vi "ENA_Recall Inst Setup.vi"(0 "Semiconductor Module Context":T1, 5 "Pins":string[](array[string])=["RF1", "RF2"], 11 "error in (no error)":errorcluster) -> (6 "Semiconductor Module Context Out":T1, 15 "error out":errorcluster)   [LabVIEW 2013]
uses:
  <vilib>/NI_TestStand_SemiconductorModule/NI_TestStand_Semiconductor_Module.lvlibp/PinMap/General/SemiconductorModuleContext.ctl
  Pin Map API/ENA Custom Instrument.lvlib
  <vilib>/NI_TestStand_SemiconductorModule/NI_TestStand_Semiconductor_Module.lvlibp
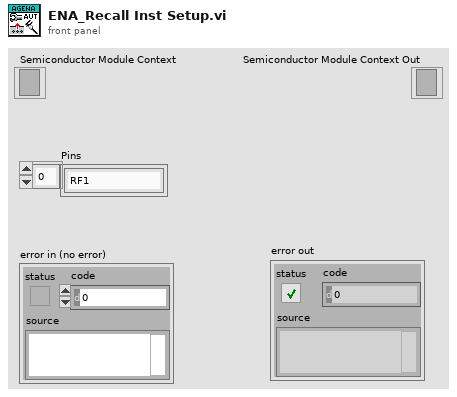
[diagram p1: front panel]
types:
  T1 = typedef "NI_TestStand_Semiconductor_Module.lvlibp/SemiconductorModuleContext.ctl" = refnum<k7>
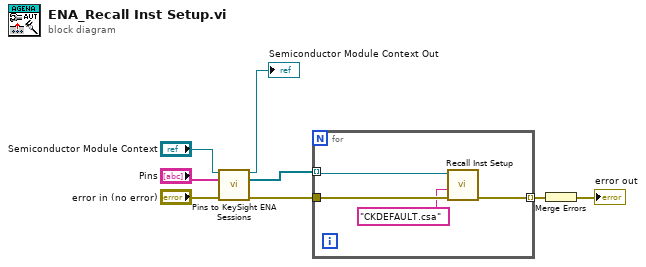
[diagram p0: block diagram]
diagram:
  n1 = call "Pins to KeySight ENA Sessions.vi"("Semiconductor Module Context"="Semiconductor Module Context", "Pins"="Pins", "error in (no error)"="error in (no error)") -> ("Semiconductor Module Context Out"=→"Semiconductor Module Context Out":T1, "Instrument Sessions"=w6:refnum<visa-resource-name>[], "error out"=w7:errorcluster)  [unwired: 8 in, 2 out]
  n2 = for {
    tunnel: w6 -> [w11] mode=indexing
    tunnel: w7 -> [w12]
    tunnel: [w9] -> w1 mode=indexing
    n3 = call "Recall Inst Setup.vi"("error in (no error)"=w12, "File Name ()"="CKDEFAULT.csa", "VISA resource name"=w11) -> ("error out"=w9:errorcluster)  [unwired: 7 in, 1 out]
  }
  n4 = Merge Errors(w1) -> (→"error out":errorcluster)
